vi "第一題.vi"() -> ()   [LabVIEW 2019]
panel:
  in  "Stop":bool
  in  "Speed":dbl(slide)=500.0 scale=100.0..500.0
  out "Knob":i32(knob)=7 scale=0.0..10.0
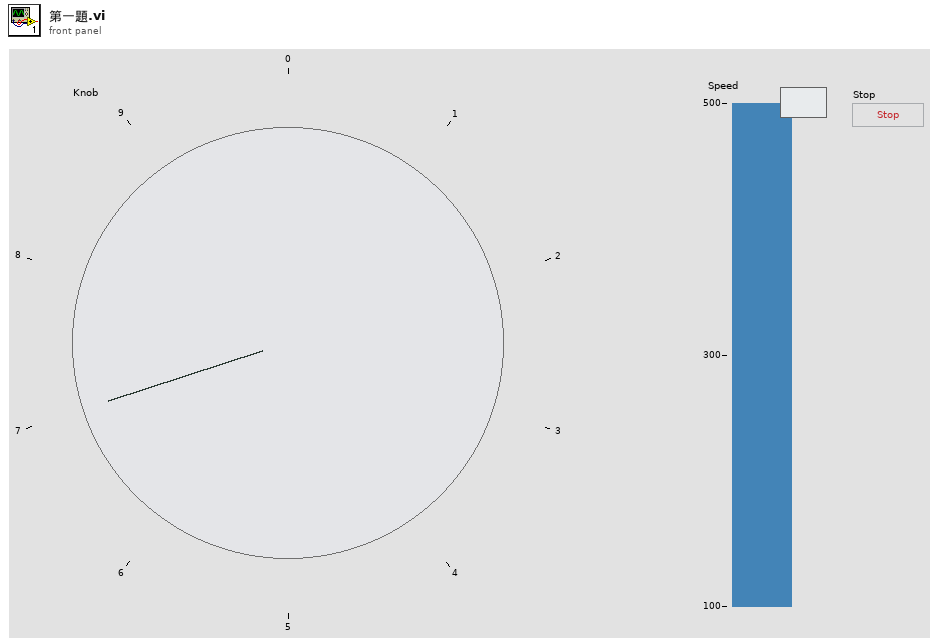
[diagram p1: front panel]
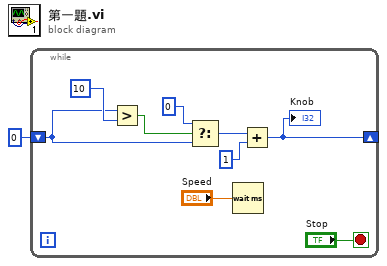
[diagram p0: block diagram]
diagram:
  n1 = while {
    shift-right: [w10] -> _
    shift-left: 0 -> [w5]
    stop <- "Stop" stop-if-true
    n2 = Greater?(x=w5, y=10) -> (0:w6:bool)
    n3 = Select(t=0, s=w6, f=w5) -> (s? t:f=w7:i32)
    n4 = Wait (ms)(milliseconds to wait="Speed") -> ()  [unwired: 1 out]
    n5 = Add(x=w7, y=1) -> (x+y=w10:i32)
    "Knob" <- w10
  }
